vi "Dialog GraphSetting (XY).vi"(11 "XYグラフref(in)":refnum<vi>) -> ()   [LabVIEW 2014]
uses:
  TypeDef/GraphSetting Appearance.ctl
  TypeDef/GraphSetting Plot.ctl
  SupportVIs/GraphSetting Scale.ctl
  TypeDef/GraphSetting DisplayFormatType.ctl
  TypeDef/GraphSetting All.ctl
  TypeDef/GraphSetting Command.ctl
  Lib/Event/Write User Event (Array).vi
  <vilib>/Utility/xml.llb/Write to XML File(string).vi
  <vilib>/Utility/xml.llb/Read From XML File(string).vi
  <vilib>/measure/NI_MABase.lvlib
  TypeDef/XYData.ctl
panel:
  out "XYグラフ":cluster{"X":dbl[], "Y":dbl[]}[](graph)
  in  "ファイル読込":bool
  in  "ファイル保存":bool
  in  "タブ制御器":enum32{"外観", "スケール", "プロット"}(tab)
  in  "外観":T1
  in  "Yスケール選択":u16(ring) items=["振幅"]
  in  "スケール(Y軸)":T2
  in  "スケール(X軸)":T2
  in  "Xスケール選択":u16(ring) items=["時間"]
  in  "プロット":T4 {"Yスケール" items=["振幅"]; "Xスケール" items=["時間"]; "プロット補間" max=5 step=1; "ポイントスタイル" max=16 step=1; "太さ" max=5 step=1; "ラインスタイル" max=4 step=1}
  in  "プロット選択":u16(ring) items=["正弦波", "プロット1"]
  in  "停止ボタン":bool
  # "スケールのスタイルとカラー"
  # "スケール係数"
  # "スケールのスタイルとカラー"
  # "スケールのスタイルとカラー"
  # "スケール係数"
  # "スケールのスタイルとカラー"
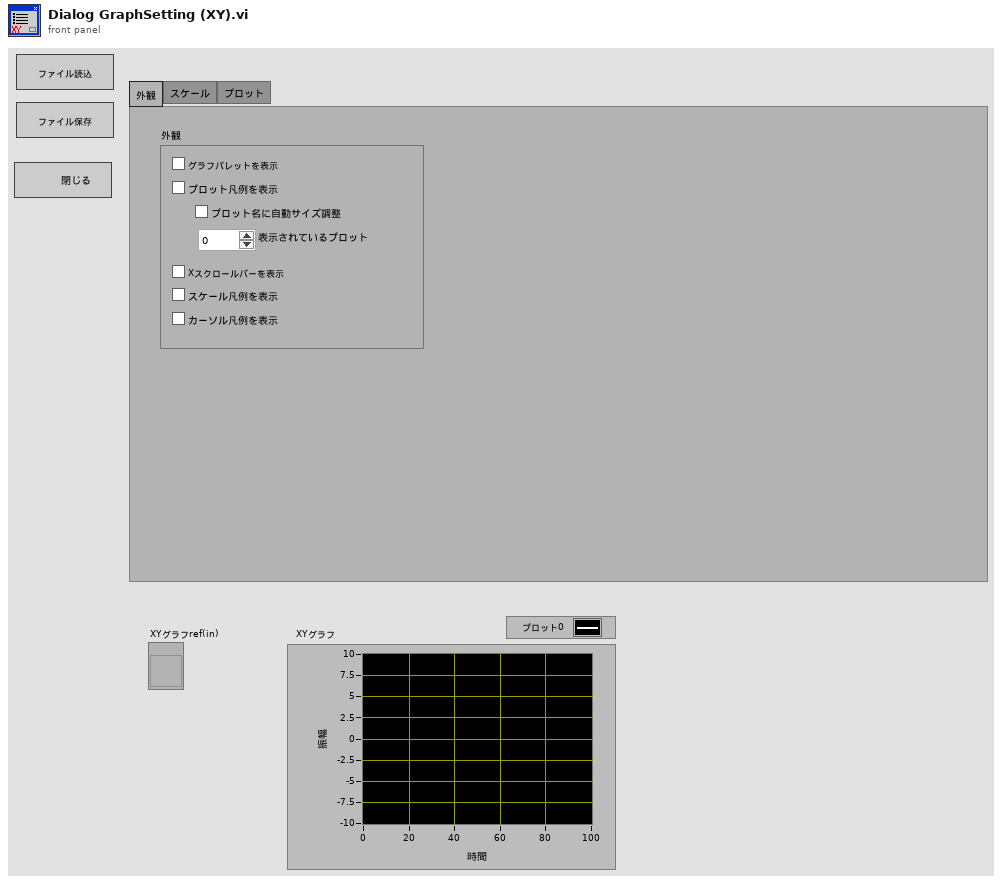
[diagram p1: front panel]
types:
  T1 = typedef "GraphSetting Appearance.ctl" = cluster{"グラフパレットを表示":bool, "プロット凡例を表示":bool, "プロット名に自動サイズ調整":bool, "表示されているプロット":u32, "Xスクロールバーを表示":bool, "スケール凡例を表示":bool, "カーソル凡例を表示":bool}
  T2 = typedef "GraphSetting Scale.ctl" = cluster{"名前":string, "スケールラベルを表示":bool, "スケールを表示":bool, "ログ":bool, "反転":bool, "自動スケール":bool, "最小":dbl, "最大":dbl, "オフセット":dbl, "乗数":dbl, "主目盛り":u32, "補助目盛り":u32, "マーカテキスト":u32, "主グリッド":u32, "補助グリッド":u32, "タイプ":T3, "小数点以下桁数":u8}
  T3 = typedef "GraphSetting DisplayFormatType.ctl" = enum8{"浮動小数点", "科学", "工学", "バイナリ", "８進数", "１６進数", "相対時間", "時間と日時", "SI"}
  T4 = typedef "GraphSetting Plot.ctl" = cluster{"名前":string, "表示":bool, "ラインスタイル":u8, "太さ":u8, "ポイントスタイル":u8, "プロット補間":u8, "ラインカラー":u32, "ポイント/塗りつぶし":u32, "Xスケール":u16, "Yスケール":u16}
  T5 = typedef "XYData.ctl" = cluster{"X":dbl[], "Y":dbl[]}
  T6 = typedef "GraphSetting All.ctl" = cluster{"外観":T1, "スケールX[]":T2[], "スケールY[]":T2[], "プロット[]":T4[]}
  T7 = typedef "GraphSetting Command.ctl" = enum16{"Get(ref->ctl)", "Set(ctl->ref)"}
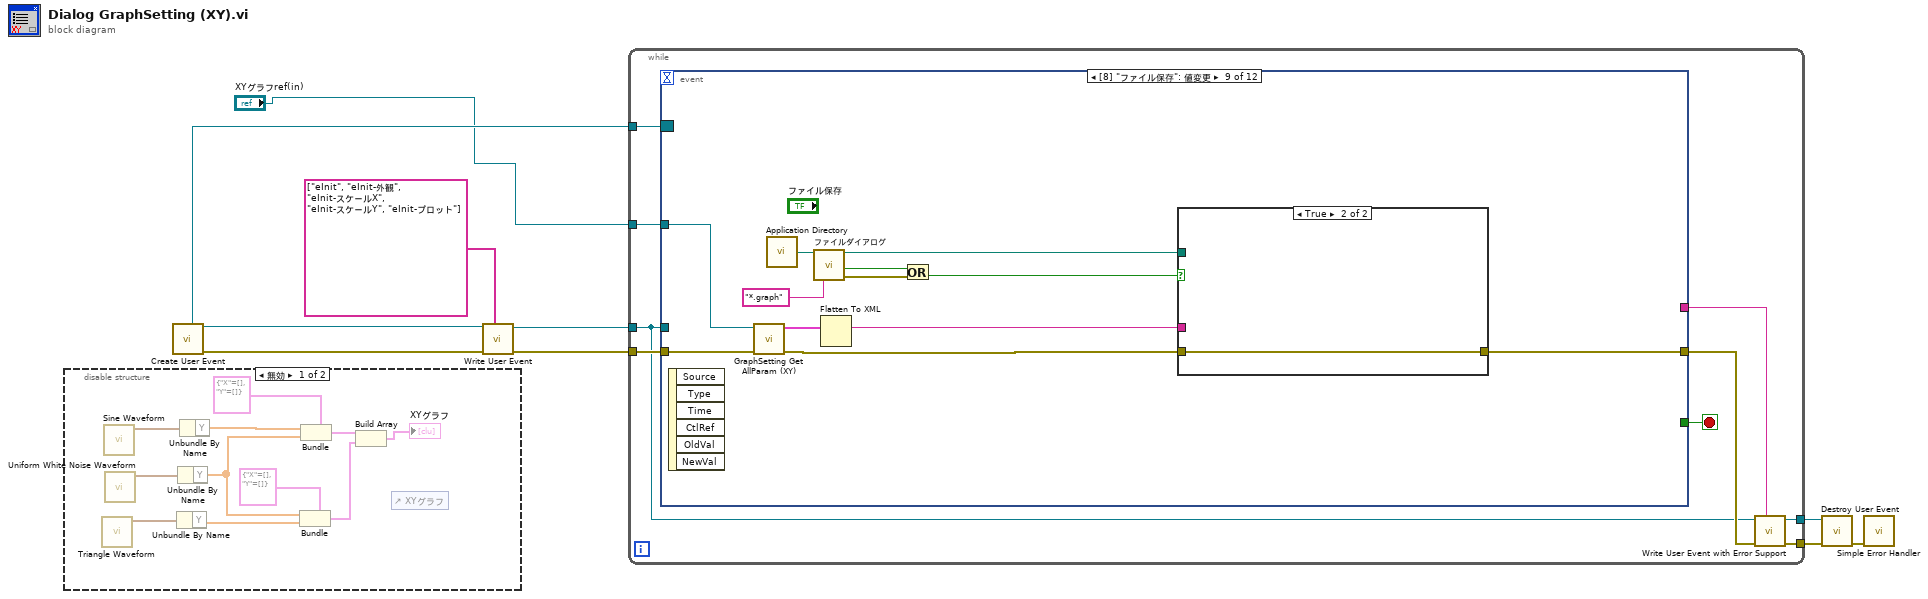
[diagram p0: block diagram]
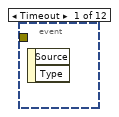
[diagram p3: hidden frame]
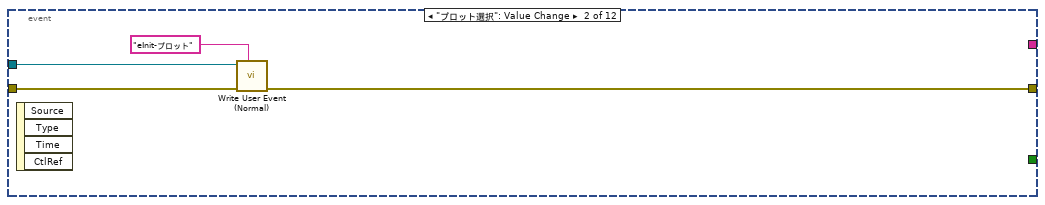
[diagram p4: hidden frame]
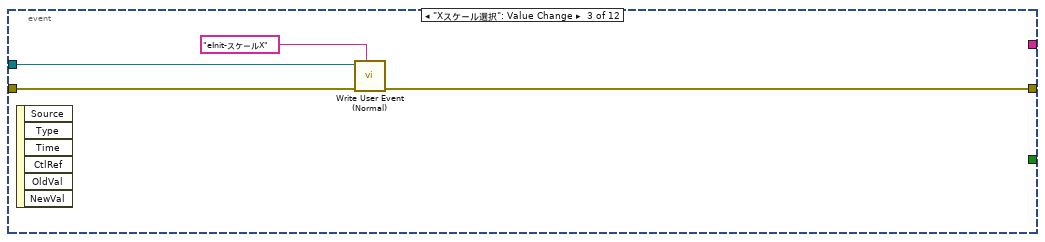
[diagram p5: hidden frame]
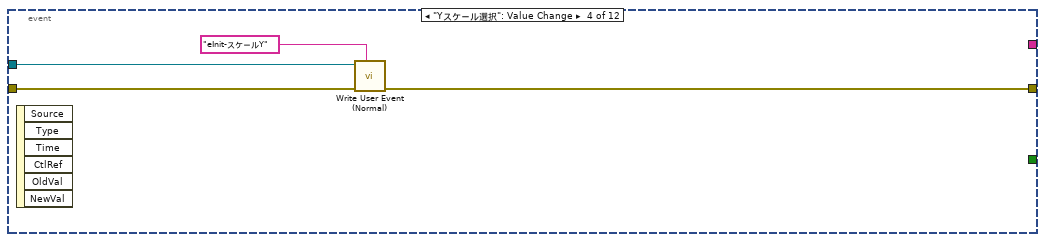
[diagram p6: hidden frame]
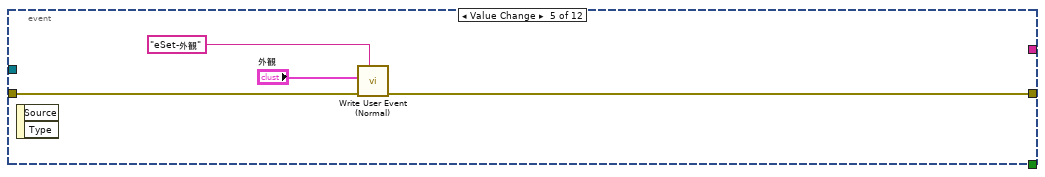
[diagram p7: hidden frame]
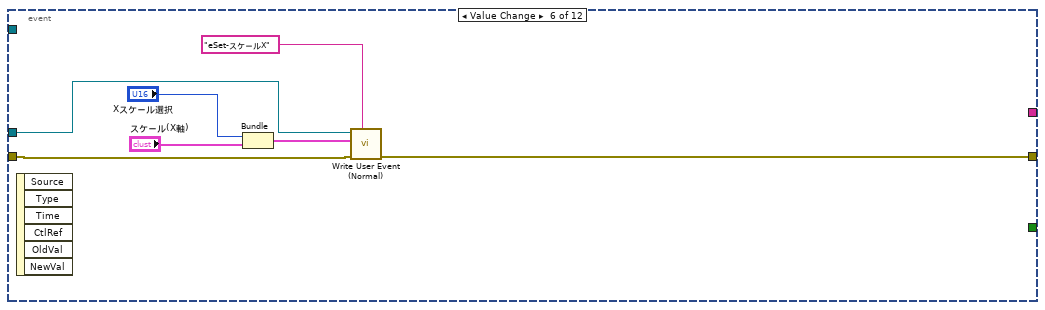
[diagram p8: hidden frame]
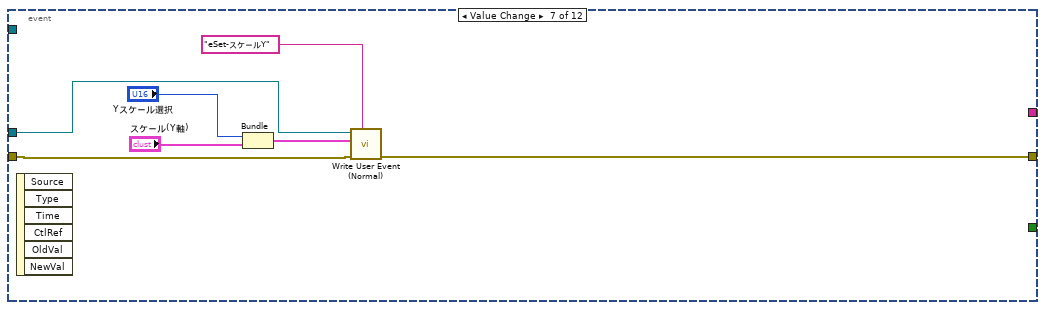
[diagram p9: hidden frame]
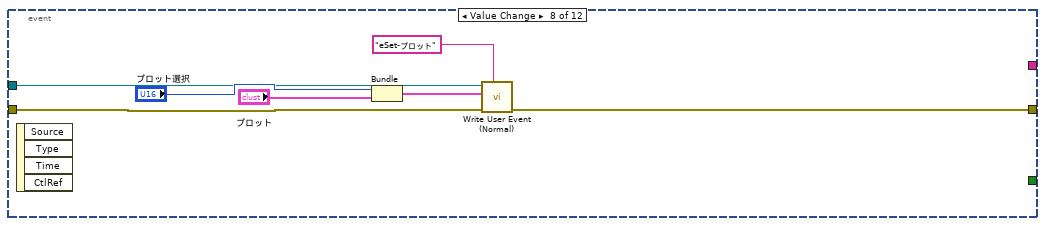
[diagram p10: hidden frame]
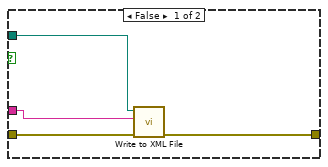
[diagram p11: hidden frame]
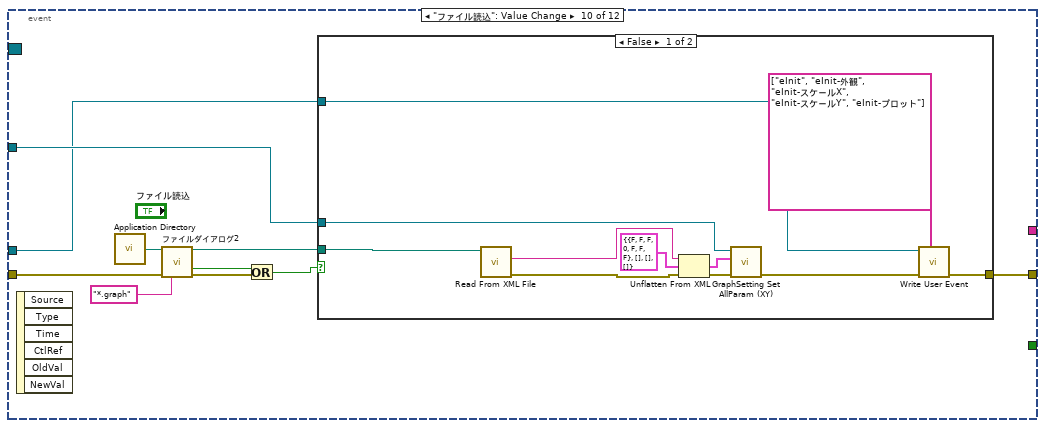
[diagram p12: hidden frame]
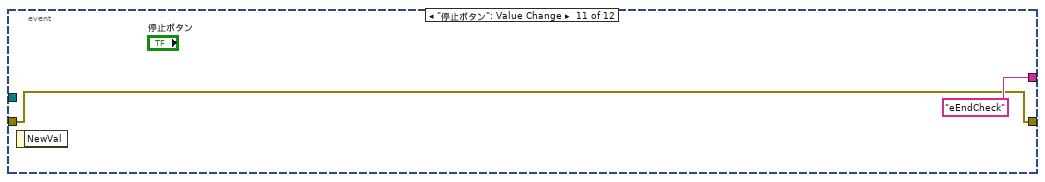
[diagram p14: hidden frame]
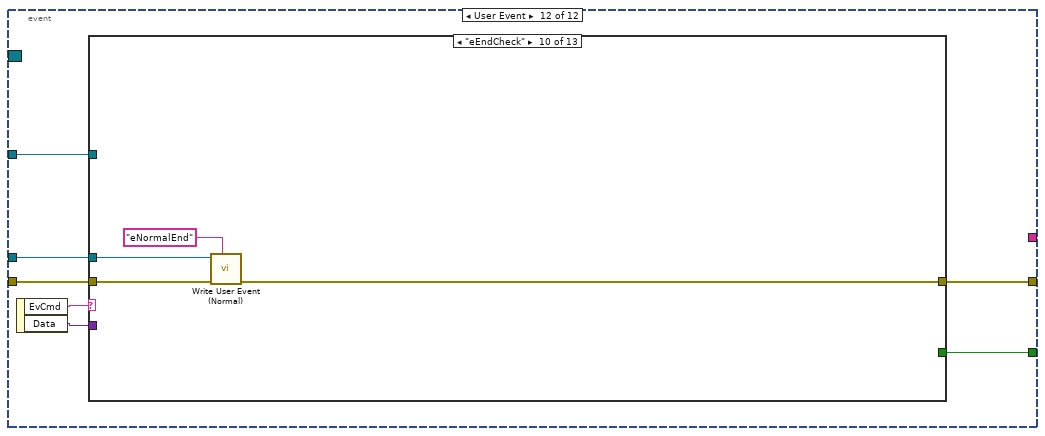
[diagram p15: hidden frame]
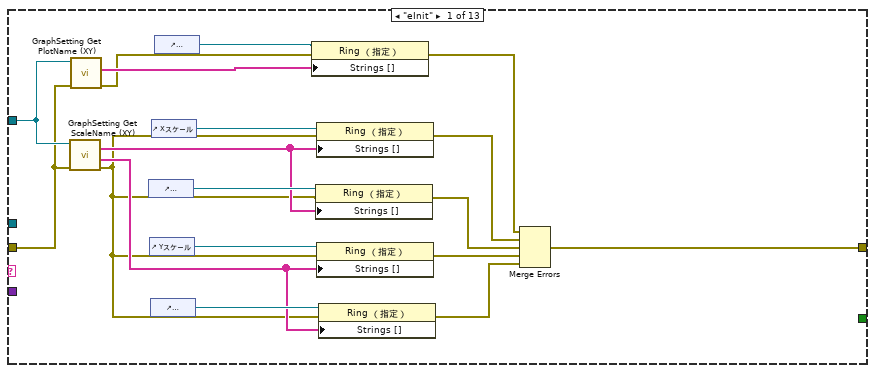
[diagram p16: hidden frame]
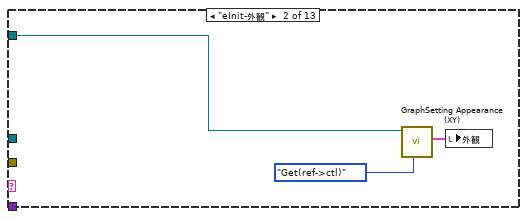
[diagram p17: hidden frame]
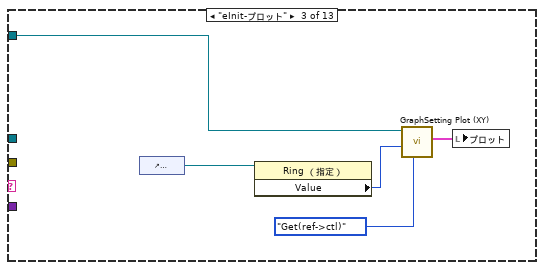
[diagram p18: hidden frame]
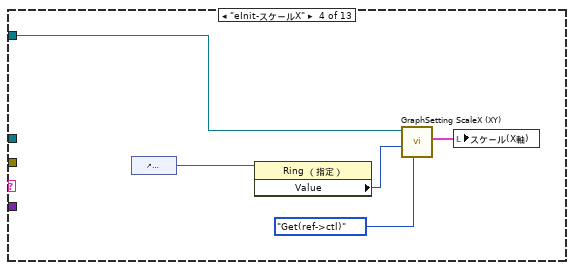
[diagram p19: hidden frame]
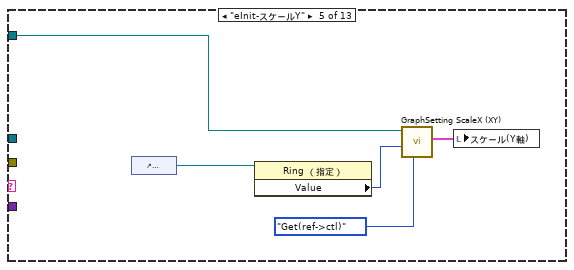
[diagram p20: hidden frame]
diagram:
  n1 = disable-structure shown="無効" {
    frame Disabled {
      n2 = call <vilib>:"Triangle Waveform.vi"() -> ("signal out"=w16:waveform(dbl))  [unwired: 10 in, 1 out]
      n3 = call <vilib>:"Sine Waveform.vi"() -> ("signal out"=w21:waveform(dbl))  [unwired: 10 in, 1 out]
      n4 = call <vilib>:"Uniform White Noise Waveform.vi"() -> ("signal out"=w17:waveform(dbl))  [unwired: 10 in, 1 out]
      n5 = Unbundle By Name(w16) -> ("Y"=w14:dbl[])
      n6 = Unbundle By Name(w17) -> ("Y"=w13:dbl[])
      n7 = Unbundle By Name(w21) -> ("Y"=w18:dbl[])
      n8 = Bundle(cluster=T5 {"X"=[], "Y"=[]} ("XYグラグデータ"), "X"=w13, "Y"=w14) -> (w11:T5)
      n9 = Bundle(cluster=T5 {"X"=[], "Y"=[]} ("XYグラグデータ"), "X"=w18, "Y"=w13) -> (w12:T5)
      n10 = Build Array(w12, w11) -> (→"XYグラフ":T5[])
      n11 = control-ref of="XYグラフ"() -> ()  [unwired: 1 out]
    }
    frame Enabled {
    }
  }
  n12 = call "Create User Event.vi"() -> ("error out"=w8:errorcluster, "User Event"=w9:refnum<user-event>, "Event Registration Refnum"=w10:refnum<event-registration>)  [unwired: 9 in]
  n13 = call-poly "Write User Event.vi"("EvCmd[]"=string[] ["eInit", "eInit-外観", "eInit-スケールX", "eInit-スケールY", "eInit-プロット"], "エラー入力（エラーなし）"=w8, "ユーザイベント入力"=w9) -> ("エラー出力"=w4:errorcluster, "ユーザイベント出力"=w5:refnum<user-event>)  [unwired: 7 in]
  n14 = while {
    tunnel: w4 -> [w29]
    tunnel: w10 -> [w30]
    tunnel: [w26] -> w7
    tunnel: w5 -> [w22]
    tunnel: "XYグラフref(in)" -> [w28]
    tunnel: [w23] -> w2
    stop <- w24 stop-if-true
    n15 = event shown="[8] \"ファイル保存\": 値変更" {
      selector: w30 -> [_ _ _ _ _ _ _ _ _ _ _ _]
      dyn-events: _ -> [_ _ _ _ _ _ _ _ _ _ _ _]
      timeout: _ -> [_ _ _ _ _ _ _ _ _ _ _ _]
      tunnel: [_ _ _ _ _ _ _ _ _ _ _ w110] -> w24
      tunnel: [_ w32 w36 w39 w43 w48 w55 w62 w75 w89 w106 w111] -> w27
      tunnel: w29 -> [_ w33 w38 w41 w44 w47 w56 w63 w72 w92 w106 w112]
      tunnel: w22 -> [_ w34 w37 w40 _ w51 w57 w64 _ w88 _ w109]
      tunnel: w28 -> [_ _ _ _ _ _ _ _ w71 w90 _ w108]
      tunnel: [_ _ _ _ _ _ _ _ _ _ "eEndCheck" _] -> w25
      event Timeout {
        n16 = event-data() -> ()  [unwired: 1 in, 2 out]
      }
      event "プロット選択": Value Change {
        n17 = event-data() -> ()  [unwired: 1 in, 4 out]
        n18 = call "Write User Event (Normal).vi"("EvCmd"="eInit-プロット", "エラー入力（エラーなし）"=w33, "ユーザイベント入力"=w34) -> ("エラー出力"=w32:errorcluster)  [unwired: 7 in, 1 out]
      }
      event "Xスケール選択": Value Change {
        n19 = event-data() -> ()  [unwired: 1 in, 6 out]
        n20 = call "Write User Event (Normal).vi"("EvCmd"="eInit-スケールX", "エラー入力（エラーなし）"=w38, "ユーザイベント入力"=w37) -> ("エラー出力"=w36:errorcluster)  [unwired: 7 in, 1 out]
      }
      event "Yスケール選択": Value Change {
        n21 = event-data() -> ()  [unwired: 1 in, 6 out]
        n22 = call "Write User Event (Normal).vi"("EvCmd"="eInit-スケールY", "エラー入力（エラーなし）"=w41, "ユーザイベント入力"=w40) -> ("エラー出力"=w39:errorcluster)  [unwired: 7 in, 1 out]
      }
      event Value Change {
        n23 = event-data() -> ()  [unwired: 1 in, 2 out]
        n24 = call "Write User Event (Normal).vi"("EvCmd"="eSet-外観", "エラー入力（エラーなし）"=w44, "データ"="外観") -> ("エラー出力"=w43:errorcluster)  [unwired: 7 in, 1 out]
      }
      event Value Change {
        n25 = event-data() -> ()  [unwired: 1 in, 6 out]
        n26 = Bundle("Xスケール選択"="Xスケール選択", "スケール(X軸)"="スケール(X軸)") -> (w52:cluster{"Xスケール選択":u16, "スケール(X軸)":T2})  [unwired: 1 in]
        n27 = call "Write User Event (Normal).vi"("EvCmd"="eSet-スケールX", "エラー入力（エラーなし）"=w47, "データ"=w52, "ユーザイベント入力"=w51) -> ("エラー出力"=w48:errorcluster)  [unwired: 6 in, 1 out]
      }
      event Value Change {
        n28 = event-data() -> ()  [unwired: 1 in, 6 out]
        n29 = Bundle("Yスケール選択"="Yスケール選択", "スケール(Y軸)"="スケール(Y軸)") -> (w58:cluster{"Yスケール選択":u16, "スケール(Y軸)":T2})  [unwired: 1 in]
        n30 = call "Write User Event (Normal).vi"("EvCmd"="eSet-スケールY", "エラー入力（エラーなし）"=w56, "データ"=w58, "ユーザイベント入力"=w57) -> ("エラー出力"=w55:errorcluster)  [unwired: 6 in, 1 out]
      }
      event Value Change {
        n31 = event-data() -> ()  [unwired: 1 in, 4 out]
        n32 = Bundle("プロット選択"="プロット選択", "プロット"="プロット") -> (w65:cluster{"プロット選択":u16, "プロット":T4})  [unwired: 1 in]
        n33 = call "Write User Event (Normal).vi"("EvCmd"="eSet-プロット", "エラー入力（エラーなし）"=w63, "データ"=w65, "ユーザイベント入力"=w64) -> ("エラー出力"=w62:errorcluster)  [unwired: 6 in, 1 out]
      }
      event "ファイル保存": Value Change {
        n34 = event-data() -> ()  [unwired: 1 in, 6 out]
        n35 = call "GraphSetting Get AllParam (XY).vi"("エラー入力（エラーなし）"=w72, "XYグラフref(in)"=w71) -> ("エラー出力"=w74:errorcluster, "クラスタ"=w73:cluster{"外観(out)":T1, T2[], T2[], T4[]})  [unwired: 8 in]
        n36 = call <vilib>:"Application Directory.vi"() -> ("Application Directory"=w78:path)
        n37 = call "ファイルダイアログ"("start path"=w78, "pattern (all files)"="*.graph") -> ("selected path"=w76:path, "cancelled"=w70:bool, "error out"=w69:errorcluster)  [unwired: 10 in, 1 out]
        n38 = Flatten To XML(anything=w73) -> (xml string=w77:string)
        n39 = Or(x=w70, y=w69) -> (x .or. y?=w68:bool)
        n40 = case shown="TRUE" w68 {
          tunnel: w76 -> [w83 _]
          tunnel: w77 -> [w82 _]
          tunnel: w74 -> [w80 w84]
          tunnel: [w81 w84] -> w75
          frame False {
            n41 = call-poly <vilib>:"Write to XML File.vi"("error in (no error)"=w80, "XML Input"=w82, "XML File Path"=w83) -> ("error out"=w81:errorcluster)  [unwired: 6 in, 2 out]
          }
          frame True {
          }
        }
      }
      event "ファイル読込": Value Change {
        n42 = event-data() -> ()  [unwired: 1 in, 6 out]
        n43 = call <vilib>:"Application Directory.vi"() -> ("Application Directory"=w94:path)
        n44 = call "ファイルダイアログ2"("start path"=w94, "error in"=w92, "pattern (all files)"="*.graph") -> ("selected path"=w91:path, "cancelled"=w87:bool, "error out"=w86:errorcluster)  [unwired: 9 in, 1 out]
        n45 = Or(x=w87, y=w86) -> (x .or. y?=w85:bool)
        n46 = case shown="FALSE" w85 {
          tunnel: w91 -> [w103 _]
          tunnel: w90 -> [w99 _]
          tunnel: [w96 _] -> w89
          tunnel: w88 -> [w98 _]
          frame False {
            n47 = call-poly <vilib>:"Read From XML File.vi"("XML File Path"=w103) -> ("error out"=w102:errorcluster, "XML Elements"=w104:string)  [unwired: 8 in, 1 out]
            n48 = Unflatten From XML(xml string=w104, type=T6 {"外観"={"グラフパレットを表示"=FALSE, "プロット凡例を表示"=FALSE, "プロット名に自動サイズ調整"=FALSE, "表示されているプロット"=0, "Xスクロールバーを表示"=FALSE, "スケール凡例を表示"=FALSE, "カーソル凡例を表示"=FALSE}, "スケールX[]"=[], "スケールY[]"=[], "プロット[]"=[]} ("出力クラスタ"), error in (no error)=w102) -> (value=w101:T6, error out=w100:errorcluster)
            n49 = call "GraphSetting Set AllParam (XY).vi"("error in (no error)"=w100, "Chartグラフパラメータ"=w101, "XYグラフref(in)"=w99) -> ("error out"=w97:errorcluster)  [unwired: 8 in]
            n50 = call-poly "Write User Event.vi"("EvCmd[]"=string[] ["eInit", "eInit-外観", "eInit-スケールX", "eInit-スケールY", "eInit-プロット"], "エラー入力（エラーなし）"=w97, "ユーザイベント入力"=w98) -> ("エラー出力"=w96:errorcluster)  [unwired: 7 in, 1 out]
          }
          frame True {
          }
        }
      }
      event "停止ボタン": Value Change {
        n51 = event-data() -> ()  [unwired: 1 in, 1 out]
      }
      event User Event {
        n52 = event-data() -> ("EvCmd"=w114:string, "Data"=w113:variant)  [unwired: 1 in]
        n53 = case shown="\"eEndCheck\"" w114 {
          selector: w114 -> [_ _ _ _ _ _ _ _ _ _ _ _ w198]
          tunnel: w113 -> [_ _ _ _ _ w155 w163 w174 w184 _ _ w197 _]
          tunnel: w112 -> [w124 _ _ _ _ w153 w165 w173 w183 w188 w192 w195 _]
          tunnel: [w115 _ _ _ _ w151 w158 w167 w177 w187 w192 _ _] -> w111
          tunnel: [_ _ _ _ _ _ _ _ _ _ TRUE TRUE _] -> w110
          tunnel: w109 -> [_ _ _ _ _ _ _ _ _ w190 _ _ _]
          tunnel: w108 -> [w127 w135 w140 w145 w150 w156 w159 w171 w181 _ _ _ _]
          frame "eInit" {
            n54 = call "GraphSetting Get ScaleName (XY).vi"("error in (no error)"=w124, "XYグラフref(in)"=w127) -> ("error out"=w121:errorcluster, "Y軸名称[]"=w123:string[], "X軸名称[]"=w130:string[])  [unwired: 7 in]
            n55 = call "GraphSetting Get PlotName (XY).vi"("error in (no error)"=w124, "XYグラフref(in)"=w127) -> ("error out"=w122:errorcluster, "プロット名称[]"=w125:string[])  [unwired: 8 in]
            n56 = control-ref of="Xスケール選択"() -> (w131:refnum<vi>)
            n57 = control-ref of="Yスケール"() -> (w128:refnum<vi>)
            n58 = control-ref of="Yスケール選択"() -> (w129:refnum<vi>)
            n59 = control-ref of="Xスケール"() -> (w132:refnum<vi>)
            n60 = control-ref of="プロット選択"() -> (w126:refnum<vi>)
            n61 = property class="Ring （指定）"(reference=w126, error in=w122, "Strings []"=w125) -> (error out=w120:errorcluster)  [unwired: 1 out]
            n62 = property class="Ring （指定）"(reference=w131, error in=w121, "Strings []"=w130) -> (error out=w118:errorcluster)  [unwired: 1 out]
            n63 = property class="Ring （指定）"(reference=w132, error in=w121, "Strings []"=w130) -> (error out=w119:errorcluster)  [unwired: 1 out]
            n64 = property class="Ring （指定）"(reference=w128, error in=w121, "Strings []"=w123) -> (error out=w117:errorcluster)  [unwired: 1 out]
            n65 = property class="Ring （指定）"(reference=w129, error in=w121, "Strings []"=w123) -> (error out=w116:errorcluster)  [unwired: 1 out]
            n66 = Merge Errors(w120, w119, w118, w117, w116) -> (w115:errorcluster)
          }
          frame "eInit-外観" {
            n67 = call "GraphSetting Appearance (XY).vi"("コマンド"=GraphSetting_Command."Get(ref->ctl)", "XYグラフref(in)"=w135) -> ("外観(out)"=w134:T1)  [unwired: 8 in, 1 out]
            n68 = local write "外観"(w134) -> ()
          }
          frame "eInit-プロット" {
            n69 = control-ref of="プロット選択"() -> (w139:refnum<vi>)
            n70 = property class="Ring （指定）"(reference=w139) -> ("Value"=w138:u16)  [unwired: 1 in, 2 out]
            n71 = call "GraphSetting Plot (XY).vi"("コマンド"=GraphSetting_Command."Get(ref->ctl)", "アクティブプロット"=w138, "XYグラフref(in)"=w140) -> ("プロット(out)"=w136:T4)  [unwired: 7 in, 1 out]
            n72 = local write "プロット"(w136) -> ()
          }
          frame "eInit-スケールX" {
            n73 = control-ref of="Xスケール選択"() -> (w144:refnum<vi>)
            n74 = property class="Ring （指定）"(reference=w144) -> ("Value"=w143:u16)  [unwired: 1 in, 2 out]
            n75 = call "GraphSetting ScaleX (XY).vi"("コマンド"=GraphSetting_Command."Get(ref->ctl)", "アクティブスケール(X)"=w143, "XYグラフref(in)"=w145) -> ("スケール(out)"=w141:T2)  [unwired: 7 in, 1 out]
            n76 = local write "スケール(X軸)"(w141) -> ()
          }
          frame "eInit-スケールY" {
            n77 = control-ref of="Yスケール選択"() -> (w149:refnum<vi>)
            n78 = property class="Ring （指定）"(reference=w149) -> ("Value"=w148:u16)  [unwired: 1 in, 2 out]
            n79 = call "GraphSetting ScaleX (XY).vi"("コマンド"=GraphSetting_Command."Get(ref->ctl)", "アクティブスケール(X)"=w148, "XYグラフref(in)"=w150) -> ("スケール(out)"=w146:T2)  [unwired: 7 in, 1 out]
            n80 = local write "スケール(Y軸)"(w146) -> ()
          }
          frame "eSet-外観" {
            n81 = Variant To Data(error in=w153, Variant=w155) -> (data=w154:T1, error out=w152:errorcluster)  [unwired: 1 in]
            n82 = call "GraphSetting Appearance (XY).vi"("コマンド"=GraphSetting_Command."Set(ctl->ref)", "error in (no error)"=w152, "外観(in)"=w154, "XYグラフref(in)"=w156) -> ("error out"=w151:errorcluster)  [unwired: 6 in, 1 out]
          }
          frame "eSet-スケールX" {
            n83 = Variant To Data(type=cluster{"Xスケール選択":u16, "スケール(X軸)":T2} {"Xスケール選択"=0, "スケール(X軸)"={"名前"="", "スケールラベルを表示"=FALSE, "スケールを表示"=FALSE, "ログ"=FALSE, "反転"=FALSE, "自動スケール"=FALSE, "最小"=0.0, "最大"=0.0, "オフセット"=0.0, "乗数"=0.0, "主目盛り"=0, "補助目盛り"=0, "マーカテキスト"=0, "主グリッド"=0, "補助グリッド"=0, "タイプ"=enum."浮動小数点", "小数点以下桁数"=0}} ("出力クラスタ"), Variant=w163) -> (data=w162:cluster{"Xスケール選択":u16, "スケール(X軸)":T2})  [unwired: 1 in, 1 out]
            n84 = Unbundle(w162) -> ("Xスケール選択"=w160:u16, "スケール(X軸)"=w161:T2)
            n85 = call "GraphSetting ScaleX (XY).vi"("コマンド"=GraphSetting_Command."Set(ctl->ref)", "error in (no error)"=w165, "アクティブスケール(X)"=w160, "スケール(in)"=w161, "XYグラフref(in)"=w159) -> ("error out"=w158:errorcluster)  [unwired: 5 in, 1 out]
          }
          frame "eSet-スケールY" {
            n86 = Variant To Data(error in=w173, type=cluster{"Xスケール選択":u16, "スケール(X軸)":T2} {"Xスケール選択"=0, "スケール(X軸)"={"名前"="", "スケールラベルを表示"=FALSE, "スケールを表示"=FALSE, "ログ"=FALSE, "反転"=FALSE, "自動スケール"=FALSE, "最小"=0.0, "最大"=0.0, "オフセット"=0.0, "乗数"=0.0, "主目盛り"=0, "補助目盛り"=0, "マーカテキスト"=0, "主グリッド"=0, "補助グリッド"=0, "タイプ"=enum."浮動小数点", "小数点以下桁数"=0}} ("出力クラスタ"), Variant=w174) -> (data=w172:cluster{"Xスケール選択":u16, "スケール(X軸)":T2}, error out=w168:errorcluster)
            n87 = Unbundle(w172) -> ("Xスケール選択"=w169:u16, "スケール(X軸)"=w170:T2)
            n88 = call "GraphSetting ScaleY (XY).vi"("コマンド"=GraphSetting_Command."Set(ctl->ref)", "error in (no error)"=w168, "アクティブスケールY"=w169, "スケール(in)"=w170, "XYグラフref(in)"=w171) -> ("error out"=w167:errorcluster)  [unwired: 5 in, 1 out]
          }
          frame "eSet-プロット" {
            n89 = Variant To Data(error in=w183, type=cluster{"プロット選択":u16, "プロット":T4} {"プロット選択"=0, "プロット"={"名前"="", "表示"=FALSE, "ラインスタイル"=0, "太さ"=0, "ポイントスタイル"=0, "プロット補間"=0, "ラインカラー"=0, "ポイント/塗りつぶし"=0, "Xスケール"=0, "Yスケール"=0}} ("出力クラスタ"), Variant=w184) -> (data=w182:cluster{"プロット選択":u16, "プロット":T4}, error out=w180:errorcluster)
            n90 = control-ref of="XYグラフ"() -> ()  [unwired: 1 out]
            n91 = Unbundle(w182) -> ("プロット選択"=w179:u16, "プロット"=w178:T4)
            n92 = call "GraphSetting Plot (XY).vi"("コマンド"=GraphSetting_Command."Set(ctl->ref)", "error in (no error)"=w180, "アクティブプロット"=w179, "プロット(in)"=w178, "XYグラフref(in)"=w181) -> ("error out"=w177:errorcluster)  [unwired: 5 in, 1 out]
          }
          frame "eEndCheck" {
            n93 = call "Write User Event (Normal).vi"("EvCmd"="eNormalEnd", "エラー入力（エラーなし）"=w188, "ユーザイベント入力"=w190) -> ("エラー出力"=w187:errorcluster)  [unwired: 7 in, 1 out]
          }
          frame "eNormalEnd" {
          }
          frame "eErrorEnd" {
            n94 = Variant To Data(error in=w195, type=errorcluster {"status"=FALSE, "code"=0, "source"=""} ("エラー定数"), Variant=w197) -> (data=w194:errorcluster)  [unwired: 1 out]
            n95 = call <vilib>:"Simple Error Handler.vi"("error in (no error)"=w194) -> ()  [unwired: 4 in, 5 out]
          }
          frame Default {
            n96 = call "DialogProgramError.vi"("エラー内容"="ユーザイベント例外" ("エラー詳細"), "エラー詳細"=w198) -> ()  [unwired: 9 in, 1 out]
          }
        }
      }
    }
    n97 = call "Write User Event with Error Support.vi"("EvCmd"=w25, "エラー入力（エラーなし）"=w27, "ユーザイベント入力"=w22) -> ("エラー出力"=w26:errorcluster, "ユーザイベント出力"=w23:refnum<user-event>)  [unwired: 7 in]
  }
  n98 = call "Destroy User Event.vi"("error in (no error)"=w7, "User Event"=w2) -> ("error out"=w6:errorcluster)  [unwired: 9 in]
  n99 = call <vilib>:"Simple Error Handler.vi"("error in (no error)"=w6) -> ()  [unwired: 4 in, 5 out]
